vi "WLAN - niVST - RFSG - Close.vi"(11 "RFSG handle":refnum<k15>="rio0") -> (0 "error out":errorcluster)   [LabVIEW 2012]
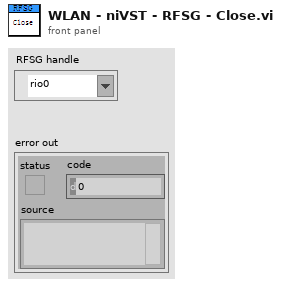
[diagram p1: front panel]
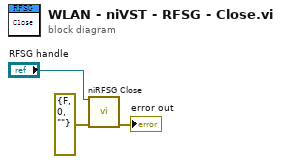
[diagram p0: block diagram]
diagram:
  n1 = call <instrlib>:"niRFSG Close.vi"("instrument handle"="RFSG handle", "error in"=errorcluster {"status"=FALSE, "code"=0, "source"=""}) -> ("error out"=→"error out":errorcluster)  [unwired: 13 in]
